vi "DrawChessboardSemiCircleSquare.vi"(0 "Bounds":T2, 1 "Skip":bool, 4 "picture in":picture, 5 "Semi Circle Square Type":T1) -> (7 "picture out":picture)   [LabVIEW 2020, in "feature_detection.lvlib"]
uses:
  feature_detection.lvlib
  Chessboard Semi Circle Square Type.ctl
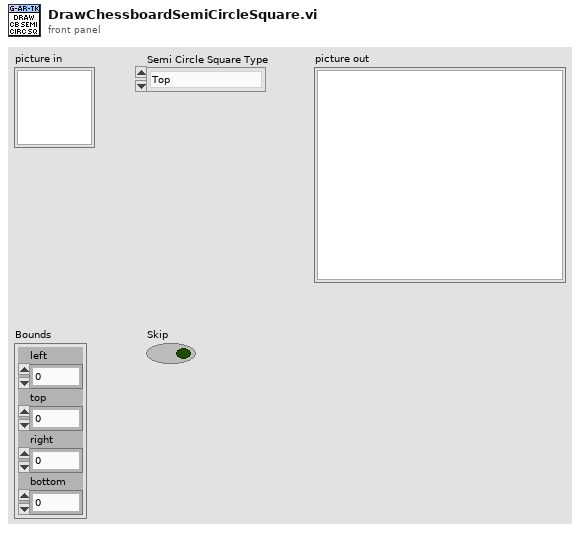
[diagram p1: front panel]
types:
  T1 = typedef "feature_detection.lvlib/Chessboard Semi Circle Square Type.ctl" = enum16{"Top", "Left", "Right", "Bottom"}
  T2 = cluster{"left":i16, "top":i16, "right":i16, "bottom":i16}
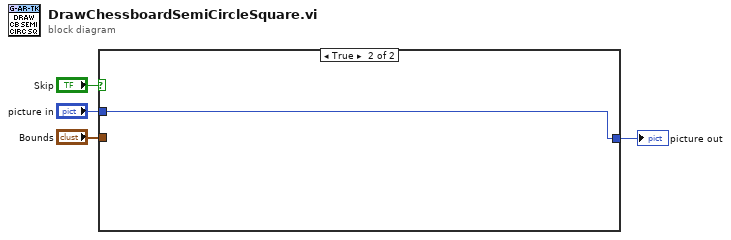
[diagram p0: block diagram]
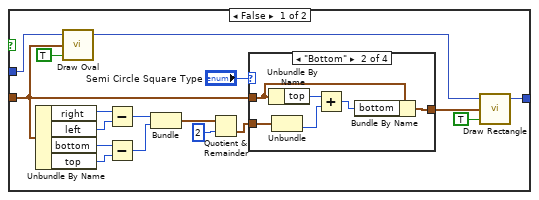
[diagram p2: hidden frame]
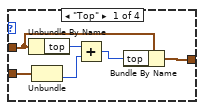
[diagram p3: hidden frame]
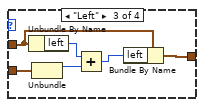
[diagram p4: hidden frame]
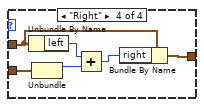
[diagram p5: hidden frame]
diagram:
  n1 = case shown="True" "Skip" {
    tunnel: [w20 w46] -> w4
    tunnel: "picture in" -> [w17 w46]
    tunnel: "Bounds" -> [w7 _]
    frame False {
      n2 = Unbundle By Name(w7) -> ("right"=w16:i16, "left"=w15:i16, "bottom"=w14:i16, "top"=w13:i16)
      n3 = call <vilib>:"Draw Oval.vi"("picture"=w17, "rect"=w7, "fill?(F)"=TRUE) -> ("new picture"=w19:picture)  [unwired: 6 in]
      n4 = Subtract(x=w16, y=w15) -> (x-y=w12:i16)
      n5 = Subtract(x=w14, y=w13) -> (x-y=w11:i16)
      n6 = Bundle(w12, w11) -> (w10:cluster{i16, i16})  [unwired: 1 in]
      n7 = Quotient & Remainder(x=w10, y=i16 2) -> (floor(x/y)=w6:cluster{i16, i16})  [unwired: 1 out]
      n8 = case shown="\"Bottom\"" "Semi Circle Square Type" {
        tunnel: w7 -> [w26 w32 w38 w44]
        tunnel: w6 -> [w25 w31 w37 w43]
        tunnel: [w27 w33 w39 w45] -> w5
        frame "Top" {
          n9 = Unbundle By Name(w26) -> ("top"=w24:i16)
          n10 = Unbundle(w25) -> (w23:i16)  [unwired: 1 out]
          n11 = Add(x=w24, y=w23) -> (x+y=w22:i16)
          n12 = Bundle By Name(cluster=w26, "top"=w22) -> (w27:T2)
        }
        frame "Bottom" {
          n13 = Unbundle By Name(w32) -> ("top"=w30:i16)
          n14 = Unbundle(w31) -> (w29:i16)  [unwired: 1 out]
          n15 = Add(x=w30, y=w29) -> (x+y=w28:i16)
          n16 = Bundle By Name(cluster=w32, "bottom"=w28) -> (w33:T2)
        }
        frame "Left" {
          n17 = Unbundle By Name(w38) -> ("left"=w36:i16)
          n18 = Unbundle(w37) -> (w34:i16)  [unwired: 1 out]
          n19 = Add(x=w36, y=w34) -> (x+y=w35:i16)
          n20 = Bundle By Name(cluster=w38, "left"=w35) -> (w39:T2)
        }
        frame "Right" {
          n21 = Unbundle By Name(w44) -> ("left"=w42:i16)
          n22 = Unbundle(w43) -> (w40:i16)  [unwired: 1 out]
          n23 = Add(x=w42, y=w40) -> (x+y=w41:i16)
          n24 = Bundle By Name(cluster=w44, "right"=w41) -> (w45:T2)
        }
      }
      n25 = call <vilib>:"Draw Rectangle.vi"("picture"=w19, "rect"=w5, "fill?(F)"=TRUE) -> ("new picture"=w20:picture)  [unwired: 6 in]
    }
    frame True {
    }
  }
  "picture out" <- w4
